vi "get_settings_cluster.vi"(8 "error in (no error)":errorcluster, 11 "GenericPlugin in":refnum<class "TrajectoryMH100122AODRAPS.lvclass">) -> (0 "error out":errorcluster, 2 "settings cluster":variant, 3 "GenericPlugin out":refnum<class "TrajectoryMH100122AODRAPS.lvclass">)   [LabVIEW 2010, in "TrajectoryMH100122AODRAPS.lvclass"]
uses:
  TrajectoryMH100122AODRAPS.lvclass
  TrajectoryMH100122AODRAPS.lvclass/TrajectoryMH100122AODRAPS.ctl
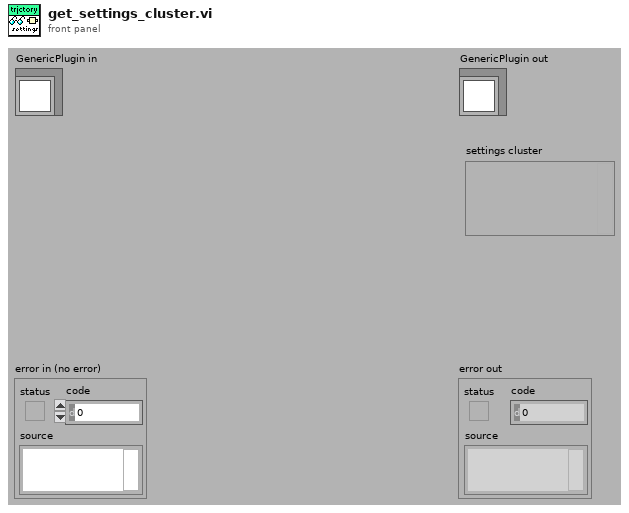
[diagram p1: front panel]
types:
  T1 = typedef "TrajectoryMH100122AODRAPS.lvclass/settings_cluster.ctl" = cluster{"no. of points":i32, "pixel dwell time":dbl[unit], "transformation factors":dbl[unit][], "2p imaging mirror switch":bool, "no. of frames":i32, "x resolution":u32, "zoom":dbl, "z angle (rotation angle, phi)":dbl[unit], "x angle (tilting angle, phi)":dbl[unit], "offset":dbl[unit][], "sub-pattern?":bool, "spiral radius":i8, "motion correction array size":u8, "y resolution":u32, "extrapolate line size":i32, "ROI color":u32, "line points color":u32, "z-step size / frame":u16, "z-offset":u16, "ROI numbering":bool, "# sub-patterns":u8, "pattern radius":u16, "# wait cycles":u16}
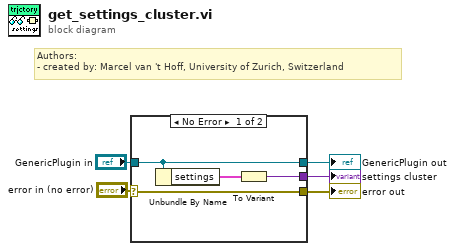
[diagram p0: block diagram]
diagram:
  # "Authors: \n- created by: Marcel van 't Hoff, University of Zurich, Switzerland"
  n1 = case shown="No Error" "error in (no error)" {
    selector: "error in (no error)" -> [w7 w10]
    tunnel: "GenericPlugin in" -> [w6 w11]
    tunnel: [w8 _] -> w3
    tunnel: [w7 w10] -> w2
    tunnel: [w6 w11] -> w1
    frame No Error {
      n2 = Unbundle By Name(w6) -> ("settings"=w9:T1)
      n3 = To Variant(anything=w9) -> (Variant=w8:variant)
    }
    frame Error {
    }
  }
  "error out" <- w2
  "GenericPlugin out" <- w1
  "settings cluster" <- w3
